vi "Set Out.vi"(8 "error in (no error)":errorcluster, 10 "Output value":refnum<class "Output Value.lvclass">, 11 "RFSoC Driver in":refnum<class "RFSoC Driver.lvclass">) -> (0 "error out":errorcluster, 3 "RFSoC Driver out":refnum<class "RFSoC Driver.lvclass">)   [LabVIEW 2019, in "RFSoC Driver.lvclass"]
uses:
  RFSoC Driver.lvclass
  <vilib>/Analysis/NI_AALBase.lvlib
  Utilities/Output Value/Output Value.lvclass
panel:
  out "data out":string
  out "Actual frequency":dbl format="%#_12pHz"
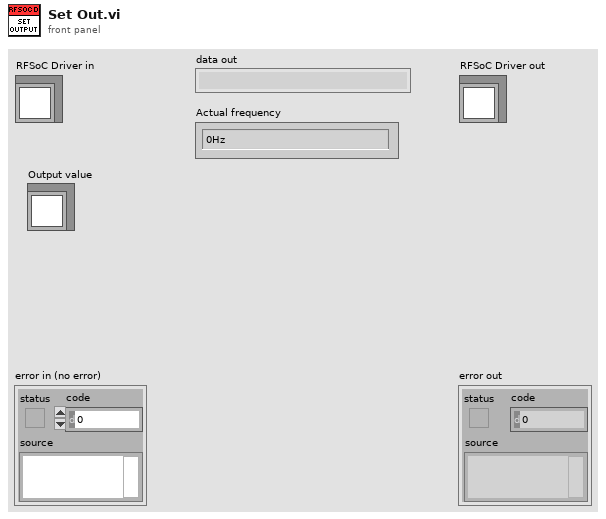
[diagram p1: front panel]
types:
  T1 = enum16{"Standard", "Buffered", "CRLF", "Immediate"}
  T2 = enum16{"big-endian, network order", "native, host order", "little-endian"}
  T3 = typedef "Pulse Parameters.ctl" = cluster{"clock rate":dbl, "Frequency":dbl, "NWaves":i32, "standard deviation":dbl, "Amplitude":dbl, "Mode":enum16{"Sine", "Pulse"}}
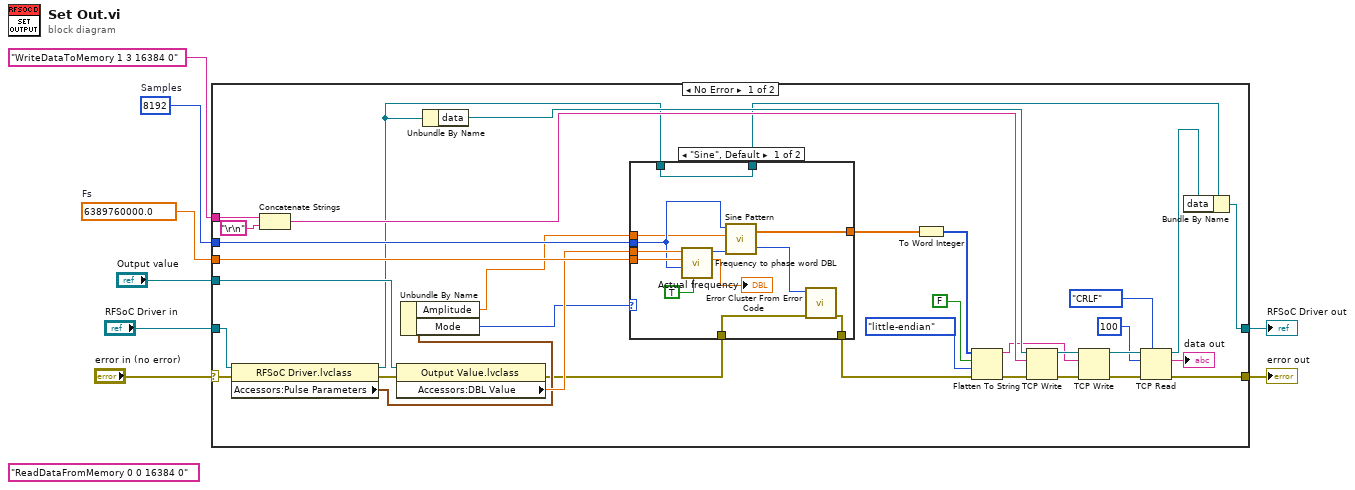
[diagram p0: block diagram]
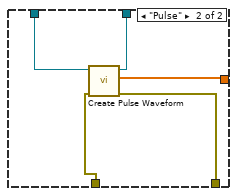
[diagram p2: hidden frame]
diagram:
  (unwired) "ReadDataFromMemory 0 0 16384 0"
  w6 = 8192  # Samples
  w7 = 6389760000.0  # Fs
  n1 = case shown="No Error" "error in (no error)" {
    selector: "error in (no error)" -> [w37 w61]
    tunnel: "Output value" -> [w42 _]
    tunnel: w7 -> [w41 _]
    tunnel: w6 -> [w39 _]
    tunnel: "RFSoC Driver in" -> [w16 w60]
    tunnel: [w22 w61] -> w3
    tunnel: [w28 w60] -> w2
    tunnel: "WriteDataToMemory 1 3 16384 0" -> [w29 _]
    frame No Error {
      n2 = property class="RFSoC Driver.lvclass"(reference=w16, error in=w37) -> (reference out=w12:refnum<class "RFSoC Driver.lvclass">, error out=w17:errorcluster, "Accessors:Pulse Parameters"=w15:T3)
      n3 = Concatenate Strings(w29, "\r\n") -> (w36:string)
      n4 = property class="Output Value.lvclass"(reference=w42, error in=w17) -> (error out=w10:errorcluster, "Accessors:DBL Value"=w40:dbl)  [unwired: 1 out]
      n5 = Unbundle By Name(w15) -> ("Amplitude"=w14:dbl, "Mode"=w13:enum16{"Sine", "Pulse"})
      n6 = Unbundle By Name(w12) -> ("data"=w30:refnum<k5>)
      n7 = case shown="\"Sine\", Default" w13 {
        tunnel: w41 -> [w54 _]
        tunnel: w40 -> [w53 _]
        tunnel: w39 -> [w50 _]
        tunnel: [w49 w58] -> w38
        tunnel: w14 -> [w47 _]
        tunnel: w12 -> [w46 w59]
        tunnel: [w46 w57] -> w11
        tunnel: w10 -> [w45 w56]
        tunnel: [w43 w55] -> w9
        frame "Sine", Default {
          n8 = call "Frequency to phase word DBL.vi"("Synchonous"=TRUE, "DDS modulus"=w50, "DDS clock"=w54, "Frequency"=w53) -> ("Actual frequency"=→"Actual frequency":dbl, "Phase word"=w51:u64)  [unwired: 6 in]
          n9 = call <vilib>:"Sine Pattern.vi"("cycles"=w51, "amplitude"=w47, "samples"=w50) -> ("error"=w44:i32, "Sinusoidal Pattern"=w49:dbl[])  [unwired: 1 in]
          n10 = call <vilib>:"Error Cluster From Error Code.vi"("error in (no error)"=w45, "error code (0)"=w44) -> ("error out"=w43:errorcluster)  [unwired: 7 in]
        }
        frame "Pulse" {
          n11 = call-dynamic "Create Pulse Waveform.vi"("error in (no error)"=w56, "RFSoC Driver in"=w59) -> ("error out"=w55:errorcluster, "Array - Numeric"=w58:dbl[], "RFSoC Driver out"=w57:refnum<class "RFSoC Driver.lvclass">)  [unwired: 7 in]
        }
      }
      n12 = To Word Integer(number=w38) -> (16bit integer=w34:i16[])
      n13 = Flatten To String(anything=w34, prepend array or string size? (T)=FALSE, byte order (0:big-endian, network order)=T2."little-endian", error in (no error)=w9) -> (data string=w25:string, error out=w31:errorcluster)  [unwired: 1 out]
      n14 = TCP Write(connection ID=w30, data in=w36, error in (no error)=w31) -> (connection ID out=w26:refnum<k5>, error out=w27:errorcluster)  [unwired: 1 in, 1 out]
      n15 = TCP Write(connection ID=w26, data in=w25, error in (no error)=w27) -> (connection ID out=w24:refnum<k5>, error out=w21:errorcluster)  [unwired: 1 in, 1 out]
      n16 = TCP Read(connection ID=w24, bytes to read=100, error in (no error)=w21, 7:T1."CRLF" ("mode (standard)")) -> (connection ID out=w23:refnum<k5>, data out=→"data out":string, error out=w22:errorcluster)  [unwired: 1 in]
      n17 = Bundle By Name(cluster=w11, "data"=w23) -> (w28:refnum<class "RFSoC Driver.lvclass">)
    }
    frame Error {
    }
  }
  "error out" <- w3
  "RFSoC Driver out" <- w2
